vi "HandleRanges.vi"(0 "reference in":refnum<class "AI.lvclass">, 11 "error in (no error)":errorcluster) -> (4 "reference out":refnum<class "AI.lvclass">, 15 "error out":errorcluster)   [LabVIEW 2019, in "AI.lvclass"]
uses:
  AI.lvclass
  AI.lvclass/AI.ctl
  AnalogComparator_class/AnalogComparator.lvclass/AnalogComparator.ctl
  AnalogComparator_class/SendToDb.vi
  AnalogComparator_class/AnalogComparator.lvclass
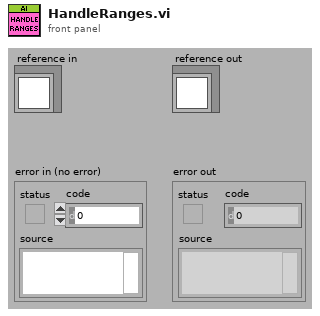
[diagram p1: front panel]
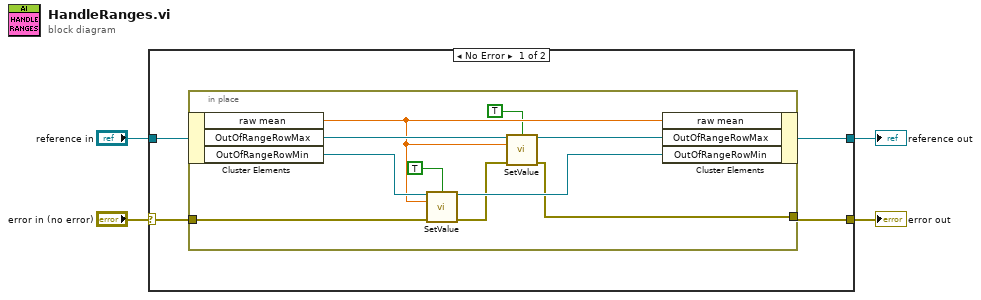
[diagram p0: block diagram]
diagram:
  n1 = case shown="No Error" "error in (no error)" {
    selector: "error in (no error)" -> [w6 w20]
    tunnel: [w5 w20] -> w3
    tunnel: [w7 w19] -> w1
    tunnel: "reference in" -> [w8 w19]
    frame No Error {
      n2 = in-place {
        in-place-border: w6 -> [w13]
        in-place-border: [w11] -> w5
        n3 = in-place-cluster #1(w8) -> ("raw mean"=w15:dbl, "OutOfRangeRowMax"=w18:refnum<class "AnalogComparator.lvclass">, "OutOfRangeRowMin"=w16:refnum<class "AnalogComparator.lvclass">)
        n4 = call "SetValue.vi"("class data in"=w16, "Enable"=TRUE, "Value"=w15, "error in (no error)"=w13) -> ("class data out"=w14:refnum<class "AnalogComparator.lvclass">, "error out"=w12:errorcluster)  [unwired: 10 in]
        n5 = call "SetValue.vi"("class data in"=w18, "Enable"=TRUE, "Value"=w15, "error in (no error)"=w12) -> ("class data out"=w17:refnum<class "AnalogComparator.lvclass">, "error out"=w11:errorcluster)  [unwired: 10 in]
        n6 = in-place-cluster #1("raw mean"=w15, "OutOfRangeRowMax"=w17, "OutOfRangeRowMin"=w14) -> (w7:refnum<class "AI.lvclass">)
      }
    }
    frame Error {
    }
  }
  "error out" <- w3
  "reference out" <- w1
